vi "test_vision.vi"(7 "error in":errorcluster) -> (27 "error out":errorcluster)   [LabVIEW 2017]
uses:
  <vilib>/vision/NI_Vision_Development_Module.lvlib
panel:
  out "Image Out":T1(plugin-control)
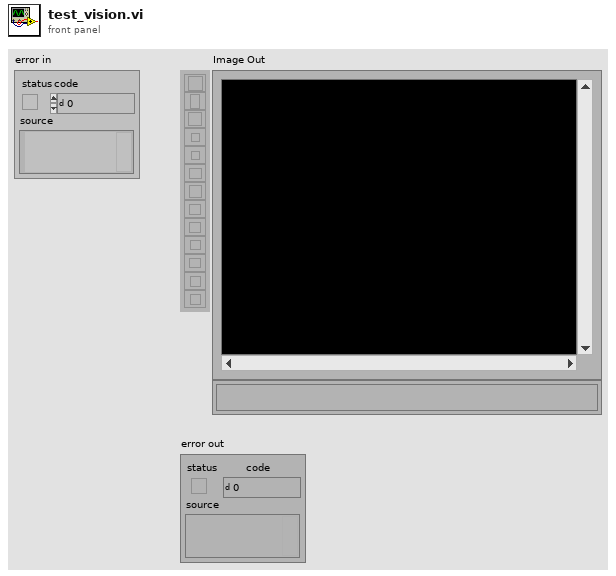
[diagram p1: front panel]
types:
  T1 = typedef "IMAQ Image.ctl" = refnum<image>
  T2 = enum32{"AutoM", "Close", "Dilate", "Erode", "Gradient", "Gradient out", "Gradient in", "Hit miss", "Open", "PClose", "POpen", "Thick", "Thin"}
  T3 = typedef "Image Type" = u32
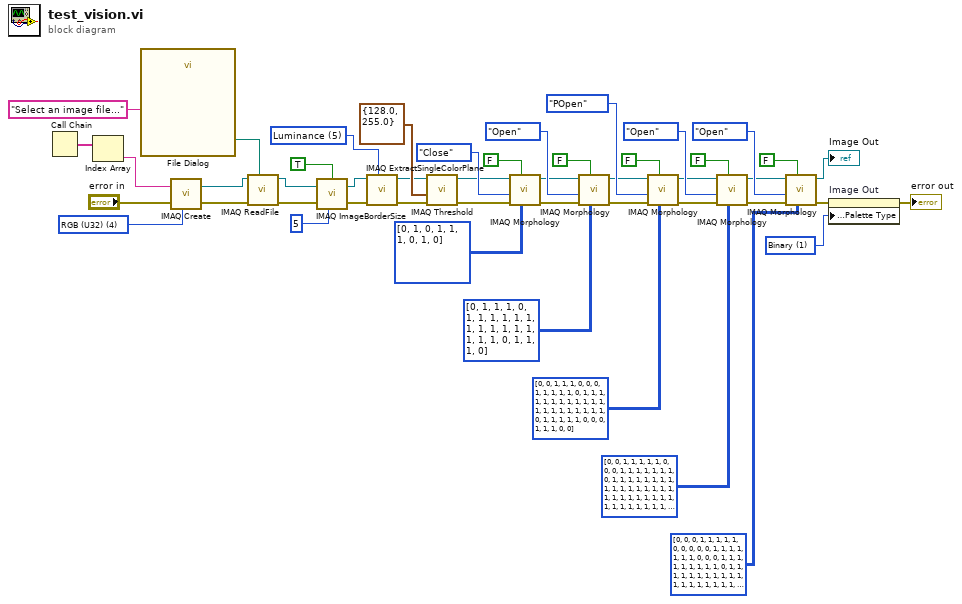
[diagram p0: block diagram]
diagram:
  w1 = u32 1 items=["Grayscale", "Binary", "Gradient", "Rainbow", "Temperature", "User Defined", "Binary 16 Bit", "Gradient 16 Bit", "Rainbow 16 Bit", "Temperature 16 Bit", "User Defined 16 Bit"] ("Palette Type")
  w35 = 5 items=["Red", "Green", "Blue", "Hue", "Saturation", "Luminance", "Value", "Intensity"] ("Color Plane")
  w40 = T3 4 items=["Grayscale (U8)", "Grayscale (I16)", "Grayscale (SGL)", "Complex (CSG)", "RGB (U32)", "HSL (U32)", "RGB (U64)", "Grayscale (U16)"] ("Image Type")
  n1 = Call Chain() -> (call chain=w44:string[])
  n2 = Index Array(array=w44) -> (element=w43:string)  [unwired: 1 in]
  n3 = call "File Dialog"("prompt"="Select an image file...") -> ("selected path"=w41:path)  [unwired: 6 in, 8 out]
  n4 = call "IMAQ Create"("Image Name"=w43, "Image Type"=w40, "error in (no error)"="error in") -> ("New Image"=w47:T1, "error out"=w46:errorcluster)  [unwired: 1 in, 1 out]
  n5 = call "IMAQ ReadFile"("File Path"=w41, "error in (no error)"=w46, "Image"=w47) -> ("error out"=w38:errorcluster, "Image Out"=w39:T1)  [unwired: 2 in, 5 out]
  n6 = call "IMAQ ImageBorderSize"("Get/Set Status? (Set)"=TRUE, "Image"=w39, "Image border size in"=5 ("Border Size"), "error in (no error)"=w38) -> ("Image Out"=w34:T1, "error out"=w33:errorcluster)  [unwired: 1 out]
  n7 = call "IMAQ ExtractSingleColorPlane"("Color Plane"=w35, "error in (no error)"=w33, "Image Src"=w34) -> ("error out"=w30:errorcluster, "Image Dst Out"=w31:T1)  [unwired: 1 in, 6 out]
  n8 = call "IMAQ Threshold"("error in (no error)"=w30, "Range"=cluster{"Lower value":sgl, "Upper value":sgl} {"Lower value"=128.0, "Upper value"=255.0}, "Image Src"=w31) -> ("error out"=w25:errorcluster, "Image Dst Out"=w26:T1)  [unwired: 3 in, 4 out]
  n9 = call "IMAQ Morphology"("Structuring Element"=i32[][] [[0, 1, 0], [1, 1, 1], [0, 1, 0]], "Square/Hexa (Square)"=FALSE, "error in (no error)"=w25, "Operation"=T2."Close", "Image Src"=w26) -> ("error out"=w20:errorcluster, "Image Dst Out"=w21:T1)  [unwired: 2 in, 3 out]
  n10 = call "IMAQ Morphology"("Structuring Element"=i32[][] [[0, 1, 1, 1, 0], [1, 1, 1, 1, 1], [1, 1, 1, 1, 1], [1, 1, 1, 1, 1], [0, 1, 1, 1, 0]], "Square/Hexa (Square)"=FALSE, "error in (no error)"=w20, "Operation"=T2."Open", "Image Src"=w21) -> ("error out"=w15:errorcluster, "Image Dst Out"=w16:T1)  [unwired: 2 in, 3 out]
  n11 = call "IMAQ Morphology"("Structuring Element"=i32[][] [[0, 0, 1, 1, 1, 0, 0], [0, 1, 1, 1, 1, 1, 0], [1, 1, 1, 1, 1, 1, 1], [1, 1, 1, 1, 1, 1, 1], [1, 1, 1, 1, 1, 1, 1], [0, 1, 1, 1, 1, 1, 0], [0, 0, 1, 1, 1, 0, 0]], "Square/Hexa (Square)"=FALSE, "error in (no error)"=w15, "Operation"=T2."POpen", "Image Src"=w16) -> ("error out"=w10:errorcluster, "Image Dst Out"=w11:T1)  [unwired: 2 in, 3 out]
  n12 = call "IMAQ Morphology"("Structuring Element"=i32[][] [[0, 0, 1, 1, 1, 1, 1, 0, 0], [0, 1, 1, 1, 1, 1, 1, 1, 0], [1, 1, 1, 1, 1, 1, 1, 1, 1], [1, 1, 1, 1, 1, 1, 1, 1, 1], [1, 1, 1, 1, 1, 1, 1, 1, 1], [1, 1, 1, 1, 1, 1, 1, 1, 1], [1, 1, 1, 1, 1, 1, 1, 1, 1], [0, 1, 1, 1, 1, 1, 1, 1, 0], [0, 0, 1, 1, 1, 1, 1, 0, 0]], "Square/Hexa (Square)"=FALSE, "error in (no error)"=w10, "Operation"=T2."Open", "Image Src"=w11) -> ("error out"=w5:errorcluster, "Image Dst Out"=w6:T1)  [unwired: 2 in, 3 out]
  n13 = call "IMAQ Morphology"("Structuring Element"=i32[][] [[0, 0, 0, 1, 1, 1, 1, 1, 0, 0, 0], [0, 0, 1, 1, 1, 1, 1, 1, 1, 0, 0], [0, 1, 1, 1, 1, 1, 1, 1, 1, 1, 0], [1, 1, 1, 1, 1, 1, 1, 1, 1, 1, 1], [1, 1, 1, 1, 1, 1, 1, 1, 1, 1, 1], [1, 1, 1, 1, 1, 1, 1, 1, 1, 1, 1], [1, 1, 1, 1, 1, 1, 1, 1, 1, 1, 1], [1, 1, 1, 1, 1, 1, 1, 1, 1, 1, 1], [0, 1, 1, 1, 1, 1, 1, 1, 1, 1, 0], [0, 0, 1, 1, 1, 1, 1, 1, 1, 0, 0], [0, 0, 0, 1, 1, 1, 1, 1, 0, 0, 0]], "Square/Hexa (Square)"=FALSE, "error in (no error)"=w5, "Operation"=T2."Open", "Image Src"=w6) -> ("error out"=w4:errorcluster, "Image Dst Out"=→"Image Out":T1)  [unwired: 2 in, 3 out]
  n14 = property on="Image Out" class="ImageControl"(error in=w4, "Palette:Palette Type"=w1) -> (error out=→"error out":errorcluster)  [unwired: 1 in, 1 out]
